vi "AddError.vi"(5 "Severity":string, 6 "Passthrough (f)":bool, 7 "Priority":u8, 8 "ErrorArray In":errorcluster[](array[cluster]), 11 "error in (no error)":errorcluster) -> (0 "ErrorArray Out":errorcluster[](array[cluster]), 3 "error out":errorcluster)   [LabVIEW 2018, in "NISTErrorLib.lvlib"]
doc: "Adds an error or warning to the error array if an error or warning occurred."
uses:
  NISTErrorLib.lvlib
panel:
  # "0 is the highest priority"
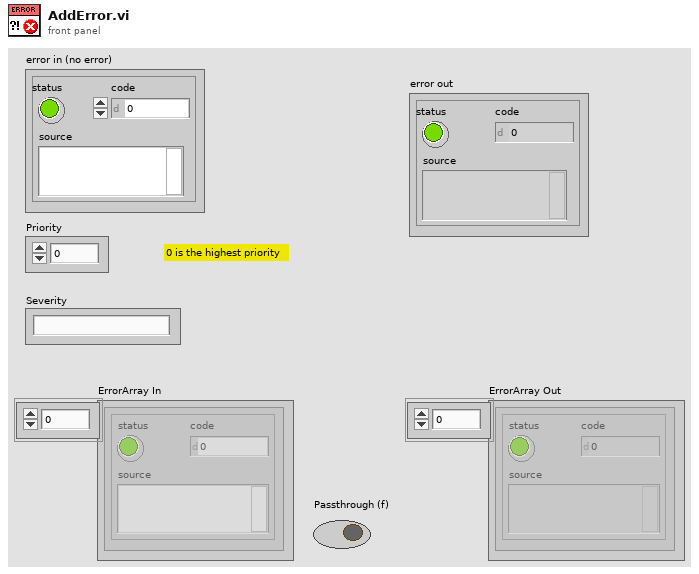
[diagram p1: front panel]
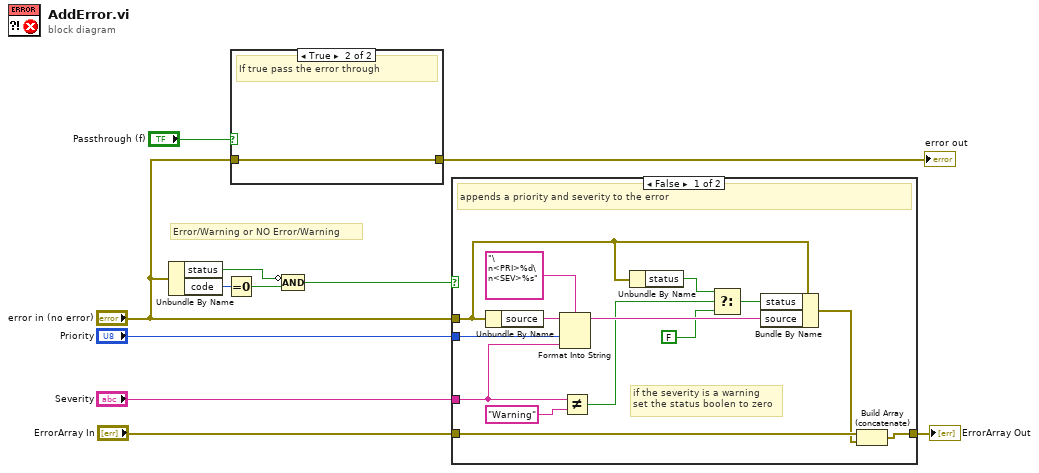
[diagram p0: block diagram]
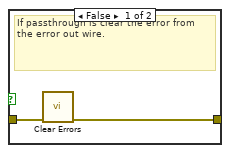
[diagram p2: hidden frame]
diagram:
  # "Error/Warning or NO Error/Warning"
  n1 = Unbundle By Name("error in (no error)") -> ("status"=w7:bool, "code"=w9:i32)
  n2 = Equal To 0?(x=w9) -> (x = 0?=w8:bool)
  n3 = case shown="True" "Passthrough (f)" {
    tunnel: "error in (no error)" -> [w13 w14]
    tunnel: [w12 w14] -> w4
    frame False {
      # "If passthrough is clear the error from \nthe error out wire."
      n4 = call <vilib>:"Clear Errors.vi"("error in (no error)"=w13) -> ("error out"=w12:errorcluster)  [unwired: 5 in, 1 out]
    }
    frame True {
      # "If true pass the error through"
    }
  }
  "error out" <- w4
  n5 = Compound Arithmetic op=AND(invert w7, w8) -> (w6:bool)
  n6 = case shown="False" w6 {
    tunnel: "Priority" -> [w26 _]
    tunnel: "Severity" -> [w21 _]
    tunnel: "ErrorArray In" -> [w24 w29]
    tunnel: [w22 w29] -> w1
    tunnel: "error in (no error)" -> [w20 _]
    frame False {
      # "if the severity is a warning\nset the status boolen to zero"
      # "appends a priority and severity to the error"
      n7 = Unbundle By Name(w20) -> ("source"=w28:string)
      n8 = Format Into String(format string="\n<PRI>%d\n<SEV>%s", initial string=w28, w26, w21) -> (resulting string=w25:string)  [unwired: 1 in, 1 out]
      n9 = Not Equal?(x=w21, y="Warning") -> (x != y?=w17:bool)
      n10 = Unbundle By Name(w20) -> ("status"=w18:bool)
      n11 = Select(t=w18, s=w17, f=FALSE) -> (s? t:f=w19:bool)
      n12 = Bundle By Name(cluster=w20, "status"=w19, "source"=w25) -> (w23:errorcluster)
      n13 = Build Array (concatenate)(w24, w23) -> (w22:errorcluster[])
    }
    frame True {
      # "no action not an error or warning"
    }
  }
  "ErrorArray Out" <- w1
